vi "遥控器测试.vi"() -> ()   [LabVIEW 2017]
uses:
  <vilib>/Instr/_visa.llb/Select Event Type.ctl
  <vilib>/Instr/_visa.llb/VISA Event Mechanism.ctl
  <vilib>/Instr/_visa.llb/VISA Flush IO Buffer Mask.ctl
  <vilib>/Instr/_visa.llb/VISA Configure Serial Port (Instr).vi
panel:
  out "右摇杆":cluster{i32[], i32[]}(graph)
  out "左摇杆":cluster{i32[], i32[]}(graph)
  out "按键":bool
  out "左-右":i32(slide) scale=-127.0..127.0
  out "前-后":i32(slide) scale=-127.0..127.0
  out "左-右 旋转":i32(slide) scale=-127.0..127.0
  out "油门":i32(slide) scale=0.0..255.0
  out "帧率":dbl(graph)
  out "单次执行时间":u32(graph)
  out "读取数据":string
  in  "停止按钮":bool
  in  "VISA resource name":refnum<visa-resource-name> caption="VISA资源名称"
  # "遥控器测试"
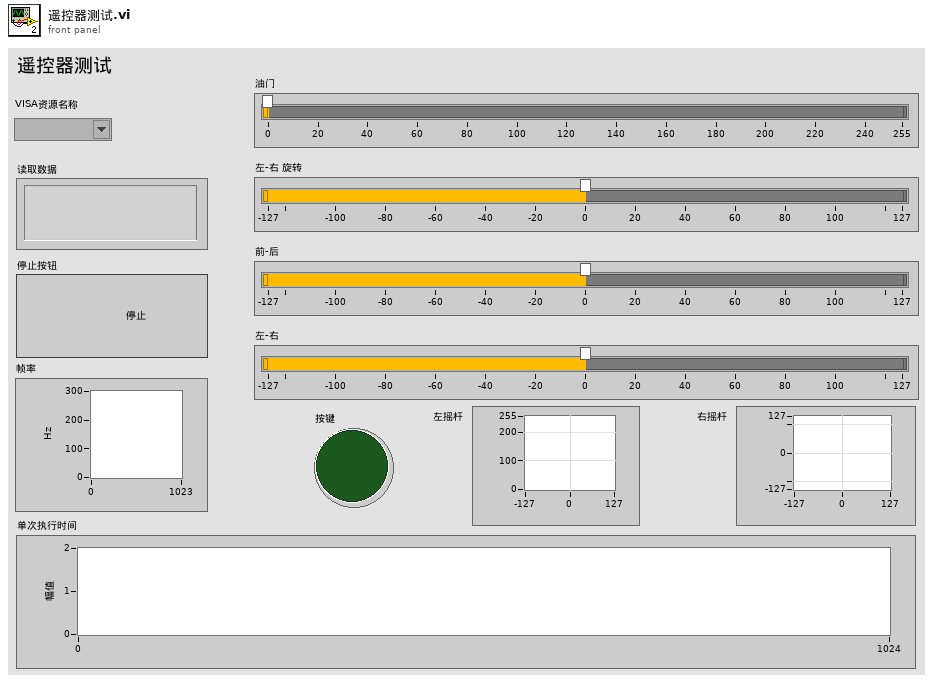
[diagram p1: front panel]
types:
  T1 = typedef "VISA Flush IO Buffer Mask.ctl" = u16
  T2 = typedef "VISA Event Mechanism.ctl" = u16
  T3 = typedef "Select Event Type.ctl" = u32
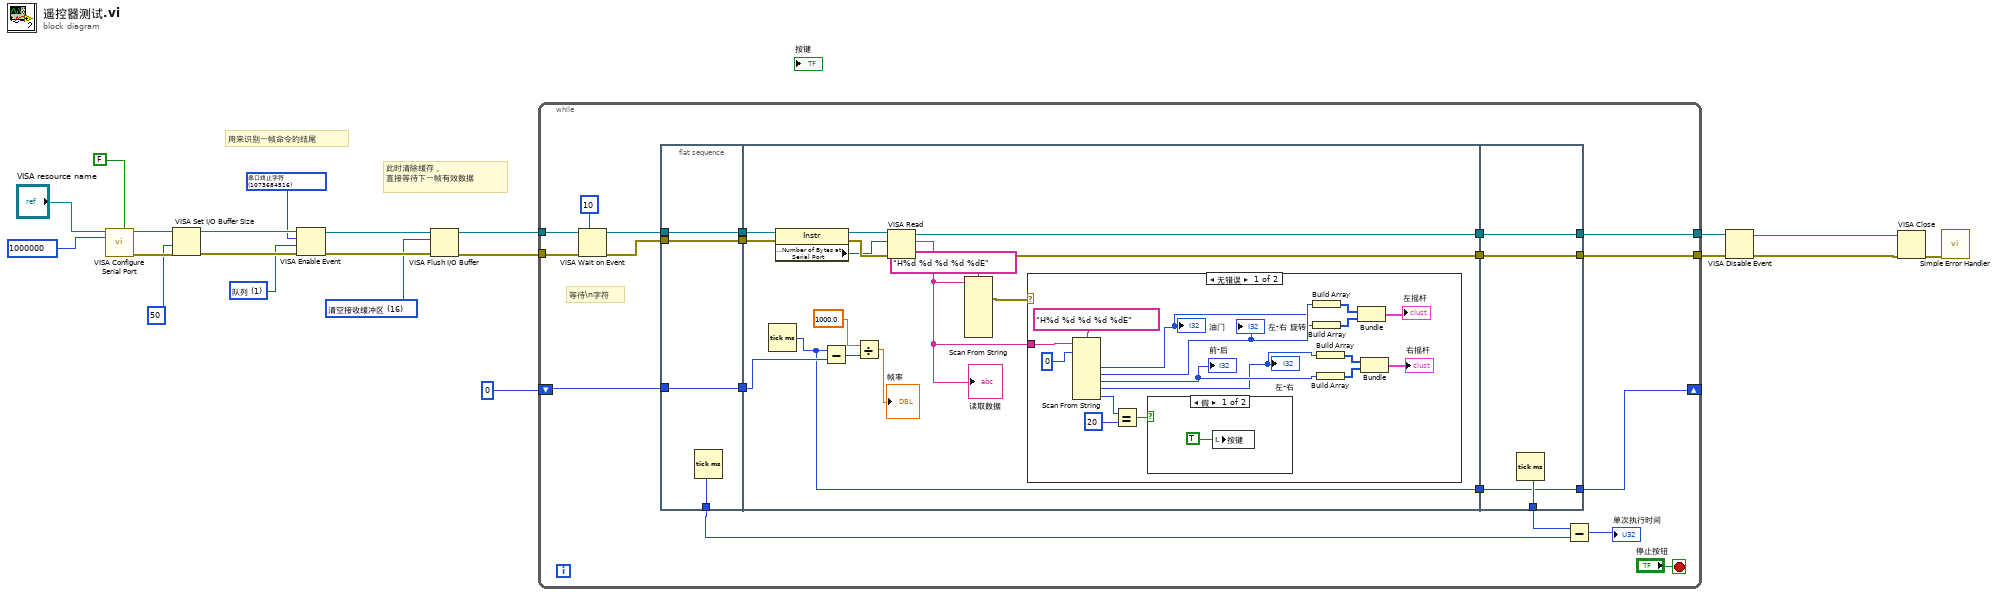
[diagram p0: block diagram]
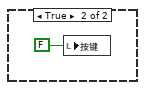
[diagram p2: hidden frame]
diagram:
  w4 = T1 16 items=["清空接收缓冲区"=16, "向设备写入传输缓冲区"=32, "清空接收缓冲区（无I/O）"=64, "清空传输缓冲区"=128] ("Mask")
  w13 = T2 1 items=["队列"=1] ("Mechanism Type")
  w14 = T3 1073684516 items=["服务请求"=1073684491, "触发"=3221168138, "清除"=1073684493, "VXI信号"=1073684512, "VXI/VME中断"=3221168161, "VXI/VME系统故障"=1073684509, "VXI/VME系统重启"=1073684510, "GPIB CIC"=1073684498, "GPIB通话"=1073684499, "GPIB侦听"=1073684500, "PXI干扰"=1073684514, "串口中断"=1073684515, "串口终止字符"=1073684516, "串口CTS"=1073684521, "串口DSR"=1073684522, "串口DCD"=1073684524, "串口RI"=1073684526, "串口字符"=1073684533, "USB中断"=1073684535, "全部启用"=1073709055] ("Event Type")
  # "用来识别一帧命令的结尾"
  # "此时清除缓存，\n直接等待下一帧有效数据"
  n1 = call-poly "VISA Configure Serial Port"("VISA resource name"="VISA resource name", "Enable Termination\nChar (T)"=FALSE ("Enable Termination\nChar (T)"), "baud rate (9600)"=u32 1000000) -> ("VISA resource name out"=w18:refnum<visa-resource-name>, "error out"=w17:errorcluster)  [unwired: 11 in]
  n2 = VISA Set I/O Buffer Size(VISA resource name=w18, size (4096)=u32 50 ("大小(4096)"), error in (no error)=w17) -> (VISA resource name out=w16:refnum<visa-resource-name>, error out=w15:errorcluster)  [unwired: 1 in]
  n3 = VISA Enable Event(8:w15, 9:w13, 10:w14, 11:w16) -> (0:w5:errorcluster, 3:w6:refnum<visa-resource-name>)
  n4 = VISA Flush I/O Buffer(VISA resource name=w6, mask (16)=w4, error in (no error)=w5) -> (VISA resource name out=w8:refnum<visa-resource-name>, error out=w7:errorcluster)
  n5 = while {
    tunnel: w8 -> [w37]
    tunnel: w7 -> [w36]
    tunnel: [w39] -> w12
    tunnel: [w38] -> w11
    shift-right: [w23] -> _
    shift-left: u32 0 -> [w26]
    stop <- "停止按钮" stop-if-true
    # "等待\\n字符"
    n6 = VISA Wait on Event(7:u32 10 ("超时(0)"), 8:w36, 11:w37) -> (0:w34:errorcluster, 3:w35:refnum<visa-resource-name>)  [unwired: 2 in, 2 out]
    n7 = flat-sequence {
      tunnel: w34 -> [w43]
      tunnel: w35 -> [w44]
      tunnel: [w44] -> w32
      tunnel: [w43] -> w31
      tunnel: [w42] -> w27
      tunnel: w26 -> [w41]
      tunnel: [w41] -> w25
      tunnel: w32 -> [w59]
      tunnel: w31 -> [w58]
      tunnel: [w49] -> w30
      tunnel: [w48] -> w29
      tunnel: w25 -> [w54]
      tunnel: [w50] -> w24
      tunnel: [w80] -> w38
      tunnel: [w81] -> w39
      tunnel: w30 -> [w81]
      tunnel: w29 -> [w80]
      tunnel: [w79] -> w28
      tunnel: w24 -> [w78]
      tunnel: [w78] -> w23
      frame #0 {
        n8 = Tick Count (ms)() -> (millisecond timer value=w42:u32)
      }
      frame #1 {
        n9 = Tick Count (ms)() -> (millisecond timer value=w50:u32)
        n10 = property class="Instr"(reference=w59, error in=w58) -> (reference out=w57:refnum<visa-resource-name>, error out=w56:errorcluster, "Serial Settings:Number of Bytes at Serial Port"=w55:u32)
        n11 = Subtract(x=w50, y=w54) -> (x-y=w53:u32)
        n12 = Divide(x=1000.0, y=w53) -> (x/y=→"帧率":dbl)
        n13 = VISA Read(VISA resource name=w57, byte count=w55, error in (no error)=w56) -> (VISA resource name out=w49:refnum<visa-resource-name>, read buffer=w47:string, error out=w48:errorcluster)  [unwired: 1 out]
        "读取数据" <- w47
        n14 = Scan From String(format string="H%d %d %d %d %dE" ("格式字符串"), input string=w47) -> (error out=w46:errorcluster)  [unwired: 12 in, 2 out]
        n15 = case shown="无错误" w46 {
          tunnel: w47 -> [w74 _]
          frame No Error {
            n16 = Scan From String(format string="H%d %d %d %d %dE" ("格式字符串"), input string=w74, initial scan location=u32 0 ("初始扫描位置")) -> (output 1=w62:i32, output 2=w63:i32, output 3=w61:i32, output 4=w60:i32, output 5=w71:i32)  [unwired: 6 in, 3 out]
            "油门" <- w62
            "左-右 旋转" <- w63
            "前-后" <- w61
            "左-右" <- w60
            n17 = Equal?(x=w71, y=20) -> (x = y?=w72:bool)
            n18 = case shown="假" w72 {
              frame False {
                n19 = local write "按键"(TRUE ("按键 1")) -> ()
              }
              frame True {
                n20 = local write "按键"(FALSE ("按键 1")) -> ()
              }
            }
            n21 = Build Array(w63) -> (w69:i32[])
            n22 = Build Array(w62) -> (w68:i32[])
            n23 = Build Array(w60) -> (w65:i32[])
            n24 = Build Array(w61) -> (w66:i32[])
            n25 = Bundle(w69, w68) -> (→"左摇杆":cluster{i32[], i32[]})  [unwired: 1 in]
            n26 = Bundle(w65, w66) -> (→"右摇杆":cluster{i32[], i32[]})  [unwired: 1 in]
          }
          frame Error {
          }
        }
      }
      frame #2 {
        n27 = Tick Count (ms)() -> (millisecond timer value=w79:u32)
      }
    }
    n28 = Subtract(x=w28, y=w27) -> (x-y=→"单次执行时间":u32)
  }
  n29 = VISA Disable Event(8:w11, 11:w12) -> (0:w1:errorcluster, 3:w2:refnum<visa-resource-name>)  [unwired: 2 in]
  n30 = VISA Close(VISA resource name=w2, error in (no error)=w1) -> (error out=w10:errorcluster)
  n31 = call <vilib>:"Simple Error Handler.vi"("error in (no error)"=w10) -> ()  [unwired: 4 in, 5 out]
